vi "VI Is Malleable.vi"(8 "error in (no error)":errorcluster, 11 "vi ref in":refnum<vi>) -> (0 "error out":errorcluster, 2 "malleable VI?":bool, 3 "vi ref out":refnum<vi>)   [LabVIEW 2017, in "Build Automation.lvlib"]
uses:
  Build Automation.lvlib
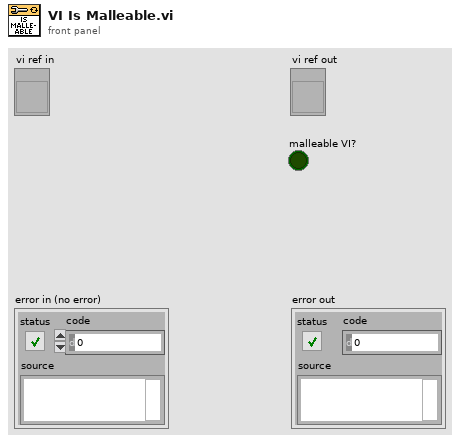
[diagram p1: front panel]
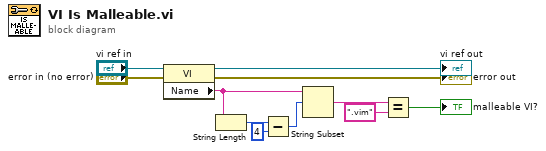
[diagram p0: block diagram]
diagram:
  n1 = property class="VI"(reference="vi ref in", error in="error in (no error)") -> (reference out=→"vi ref out":refnum<vi>, error out=→"error out":errorcluster, "Name"=w11:string)
  n2 = String Length(string=w11) -> (length=w10:i32)
  n3 = Subtract(x=w10, y=4) -> (x-y=w7:i32)
  n4 = String Subset(string=w11, offset (0)=w7) -> (substring=w9:string)  [unwired: 1 in]
  n5 = Equal?(x=w9, y=".vim") -> (x = y?=→"malleable VI?":bool)
